vi "APS absolute move.vi"(8 "error in (no error)":errorcluster caption="错误输入（无错误）", 9 "Max_Speed":i32, 10 "Distance":i32, 11 "Axis_ID":i32) -> (0 "error out":errorcluster caption="错误输出", 3 "function return":i32)   [LabVIEW 2017]
doc: "I32 FNTYPE APS_relative_move( I32 Axis_ID, I32 Distance, I32 Max_Speed );"
uses:
  APS168.lvlib
  Global/global.vi
  APS168.dll
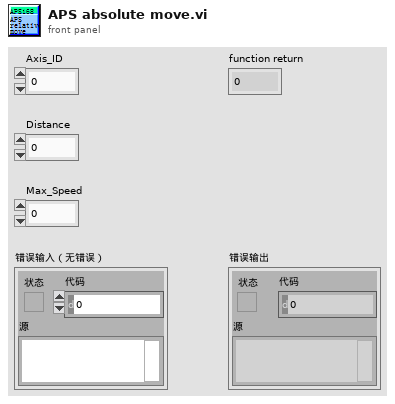
[diagram p1: front panel]
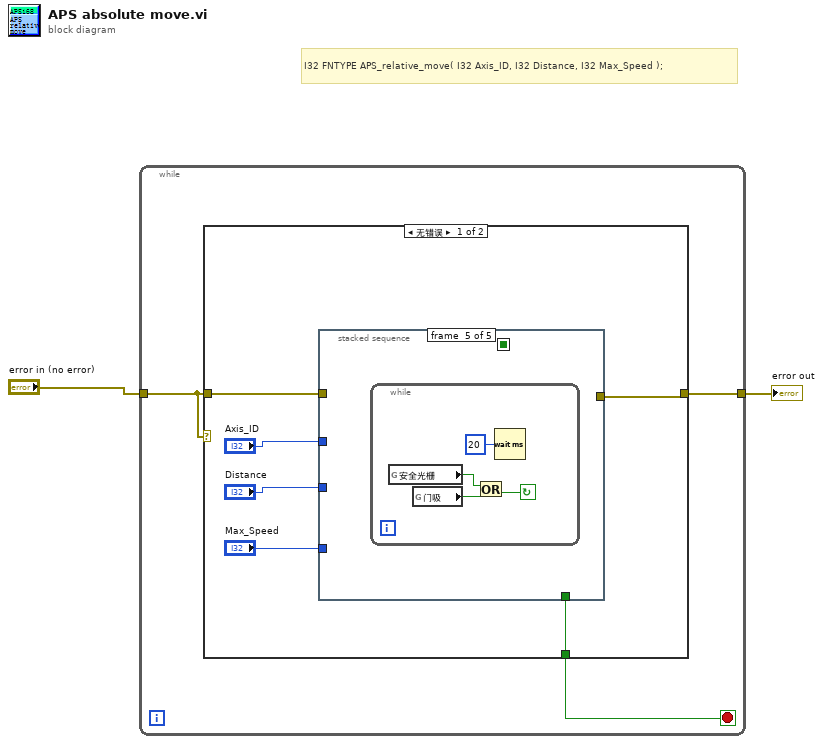
[diagram p0: block diagram]
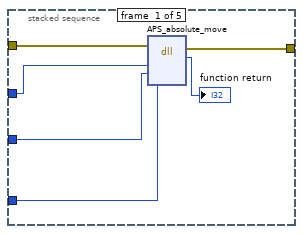
[diagram p2: hidden frame]
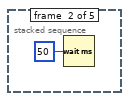
[diagram p3: hidden frame]
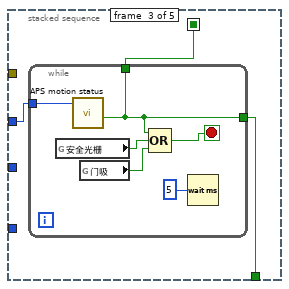
[diagram p4: hidden frame]
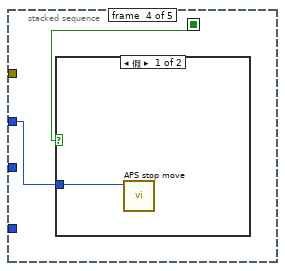
[diagram p5: hidden frame]
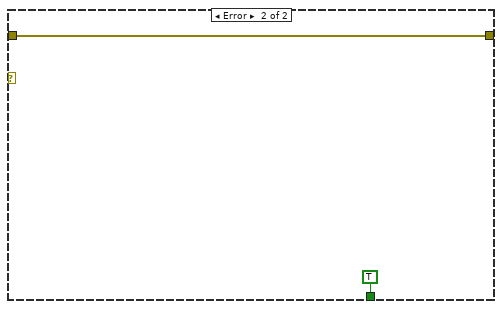
[diagram p7: hidden frame]
diagram:
  # "I32 FNTYPE APS_relative_move( I32 Axis_ID, I32 Distance, I32 Max_Speed );"
  n1 = while {
    tunnel: [w5] -> w2
    tunnel: "error in (no error)" -> [w4]
    stop <- w3 stop-if-true
    n2 = case shown="无错误" w4 {
      tunnel: [w6 w36] -> w5
      tunnel: w4 -> [w11 w36]
      tunnel: [w7 TRUE ("x与y?")] -> w3
      frame No Error {
        n3 = stacked-sequence {
          seq-local: [_ _ w20 _ _] -> [_ _ _ w29 _]
          tunnel: [_ _ w21 _ _] -> w7
          tunnel: w11 -> [w17 _ _ _ _]
          tunnel: "Axis_ID" -> [w14 _ w19 w28 _]
          tunnel: "Distance" -> [w13 _ _ _ _]
          tunnel: "Max_Speed" -> [w12 _ _ _ _]
          tunnel: [w16 _ _ _ _] -> w6
          frame #0 {
            n4 = dll-call lib="PTH2Gabs E迈治LV范例testSubVIsADLINKMotion204cAPS168.*" fn="APS_absolute_move"(error in=w17, "Axis_ID"=w14, "Position"=w13, "Max_Speed"=w12) -> (error out=w16:errorcluster, "return type"=→"function return":i32)  [unwired: 5 in, 1 out]
          }
          frame #1 {
            n5 = Wait (ms)(milliseconds to wait=u32 50 ("等待时间（毫秒）")) -> ()  [unwired: 1 out]
          }
          frame #2 {
            n6 = while {
              tunnel: w19 -> [w26]
              tunnel: [w23] -> w21
              tunnel: [w23] -> w20
              stop <- w25 stop-if-true
              n7 = global read "global.vi" "安全光栅"() -> (w24:bool)
              n8 = call "APS motion status.vi"("Axis_ID"=w26) -> ("x与y?"=w23:bool)  [unwired: 9 in, 1 out]
              n9 = global read "global.vi" "门吸"() -> (w22:bool)
              n10 = Compound Arithmetic op=OR(w23, w24, w22) -> (w25:bool)
              n11 = Wait (ms)(milliseconds to wait=u32 5 ("等待时间（毫秒）")) -> ()  [unwired: 1 out]
            }
          }
          frame #3 {
            n12 = case shown="假" w29 {
              tunnel: w28 -> [w30 _]
              frame False {
                n13 = call "APS stop move.vi"("Axis_ID"=w30) -> ()  [unwired: 9 in, 2 out]
              }
              frame True {
              }
            }
          }
          frame #4 {
            n14 = while {
              stop <- w31 continue-if-true
              n15 = global read "global.vi" "安全光栅"() -> (w32:bool)
              n16 = global read "global.vi" "门吸"() -> (w33:bool)
              n17 = Or(x=w32, y=w33) -> (x .or. y?=w31:bool)
              n18 = Wait (ms)(milliseconds to wait=u32 20 ("等待时间（毫秒）")) -> ()  [unwired: 1 out]
            }
          }
        }
      }
      frame Error {
      }
    }
  }
  "error out" <- w2
